vi "Power Fit Intervals.vi"   [LabVIEW 2018, in "NI_AALPro.lvlib"]
doc: "Calculates statistical intervals of the best power fit for a data set (<B>X</B>, <B>Y</B>). You must manually select the polymorphic instance to use."
uses:
  <vilib>/Analysis/NI_AALPro.lvlib
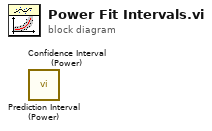
[diagram p0: block diagram]
diagram:
  n1 = call "Prediction Interval (Power).vi"() -> ()  [unwired: 13 in, 3 out]
  n2 = call "Confidence Interval (Power).vi"() -> ()  [unwired: 11 in, 5 out]
